vi "testAESEncryption-ECB-256.vi"(8 "error in (no error)":errorcluster, 11 "TestCase in":refnum<class "TestAES.lvclass">) -> (0 "error out":errorcluster, 3 "TestCase out":refnum<class "TestAES.lvclass">)   [LabVIEW 2021, in "TestAES.lvclass"]
uses:
  TestAES.lvclass
  TestAES.lvclass/TestAES.ctl
  <vilib>/addons/_JKI Toolkits/VI Tester/TestCase.llb/TestCase.lvclass
  Symmetric Encryption/dotNET Crypto Symmetric Encryption.lvlib
  <vilib>/Wiresmith Technology/VITAC (VI Tester Advanced Comparisons)/VITAC.lvlib
  C:/Program Files (x86)/National Instruments/LabVIEW 2021/vi.lib/addons/_JKI Toolkits/VI Tester/TestCase.llb/TestCase.lvclass
  C:/LabVIEW Working Directory/labview-keystore/Unit Tests/TestAES/TestAES.lvclass
panel:
  out "Key (hex)":string="01234567890"
  out "Expected ciphertext (hex)":string
  out "Actual ciphertext (hex)":string
  out "Expected ciphertext":string
  out "Plaintext in":string="Hello, World!"
  out "Actual ciphertext":string
  out "Key":string="01234567890"
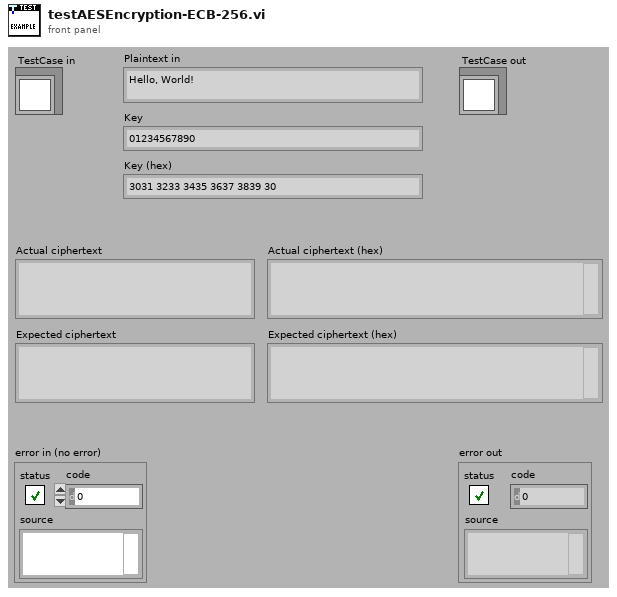
[diagram p1: front panel]
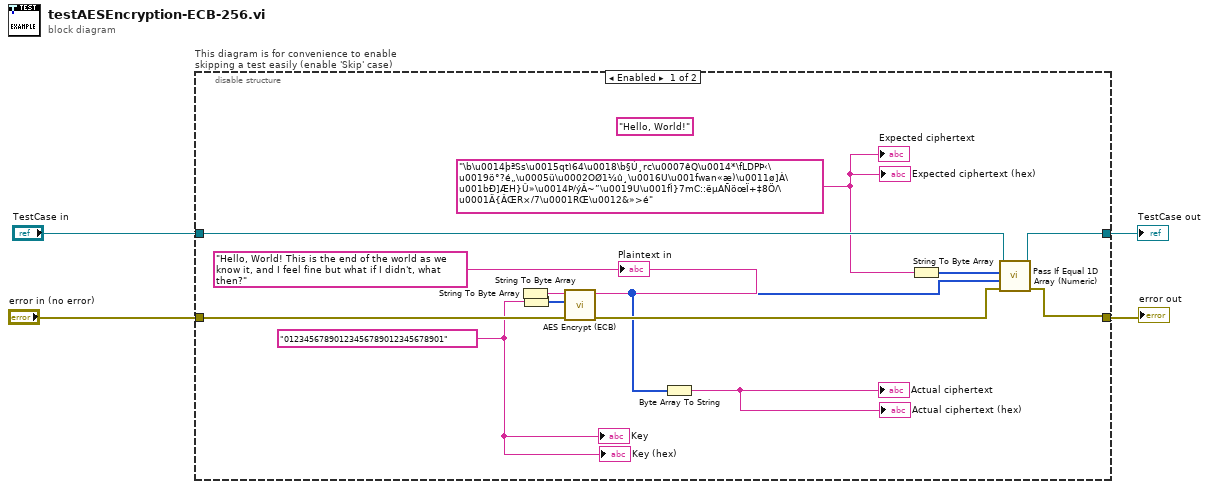
[diagram p0: block diagram]
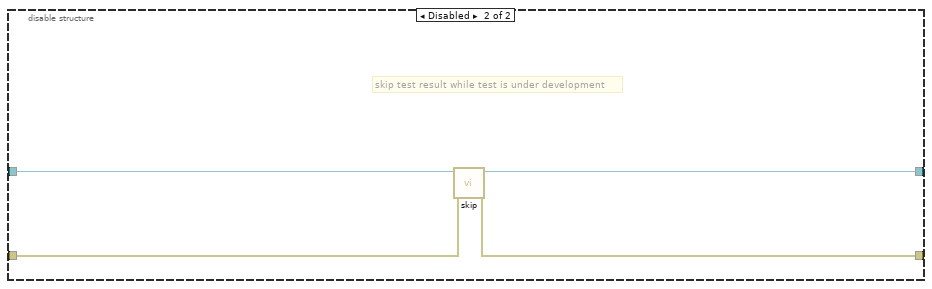
[diagram p2: hidden frame]
diagram:
  n1 = disable-structure "This diagram is for convenience to enable skipping a test easily (enable 'Skip' case)" shown="Enabled" {
    disable-tunnel: "TestCase in" -> [w17 w21]
    disable-tunnel: [w16 w19] -> w1
    disable-tunnel: [w15 w20] -> w3
    disable-tunnel: "error in (no error)" -> [w14 w18]
    frame Enabled {
      w11 = "\b\u0014þªSs\u0015qtì64\u0018\b§Ú¸rc\u0007êQ\u0014*\fLDPÞ‹\u0019ö°?é„\u0005ü\u0002OØ1¼û¸\u0016U\u001fwan«æ)\u0011ø]À\u001bÐ]ÆH}Û»\u0014Þ/ýÂ~”\u0019U\u001fÌ}7mC::ëµAÑöœÏ+‡8Ö/\u0001Ä{ÂŒR×/7\u0001RŒ\u0012&»>é" ("Plaintext in")
      (unwired) "Hello, World!" ("Plaintext in")
      w10 = "01234567890123456789012345678901" ("Key")
      w12 = "Hello, World! This is the end of the world as we know it, and I feel fine but what if I didn't, what then?" ("Plaintext in")
      n2 = String To Byte Array(string=w12) -> (unsigned byte array=w8:u8[])
      n3 = String To Byte Array(string=w10) -> (unsigned byte array=w7:u8[])
      n4 = call "AES Encrypt (ECB).vi"("error in (no error)"=w14, "Key"=w7, "Raw data in"=w8) -> ("error out"=w13:errorcluster, "Encrypted data out"=w5:u8[])  [unwired: 7 in]
      n5 = Byte Array To String(unsigned byte array=w5) -> (string=→"Actual ciphertext" →"Actual ciphertext (hex)":string)
      n6 = String To Byte Array(string=w11) -> (unsigned byte array=w9:u8[])
      n7 = call <vilib>:"Pass If Equal 1D Array (Numeric).vi"("error in (no error)"=w13, "actual"=w5, "expected"=w9, "TestCase in"=w17) -> ("error out"=w15:errorcluster, "TestCase out"=w16:refnum<class "TestAES.lvclass">)  [unwired: 6 in]
      "Key" <- w10
      "Plaintext in" <- w12
      "Expected ciphertext" <- w11
      "Expected ciphertext (hex)" <- w11
      "Key (hex)" <- w10
    }
    frame Disabled {
      # "skip test result while test is under development"
      n8 = call <vilib>:"skip.vi"("error in (no error)"=w18, "TestCase in"=w21) -> ("error out"=w20:errorcluster, "TestCase out"=w19:refnum<class "TestAES.lvclass">)  [unwired: 8 in]
    }
  }
  "error out" <- w3
  "TestCase out" <- w1
